vi "Organize new Comics.vi"() -> ()   [LabVIEW 2024]
uses:
  TypeDefs/comic--cluster.ctl
  TypeDefs/comics.reply--cluster.ctl
  <vilib>/addons/_JKI.lib/Serialization/JSON/JKI JSON Serialization.lvlib
panel:
  out "error out":errorcluster
  out "missing series":string[](array[string])
  out "current comic":string
  in  "comic repo path":path
  in  "comic data path":path
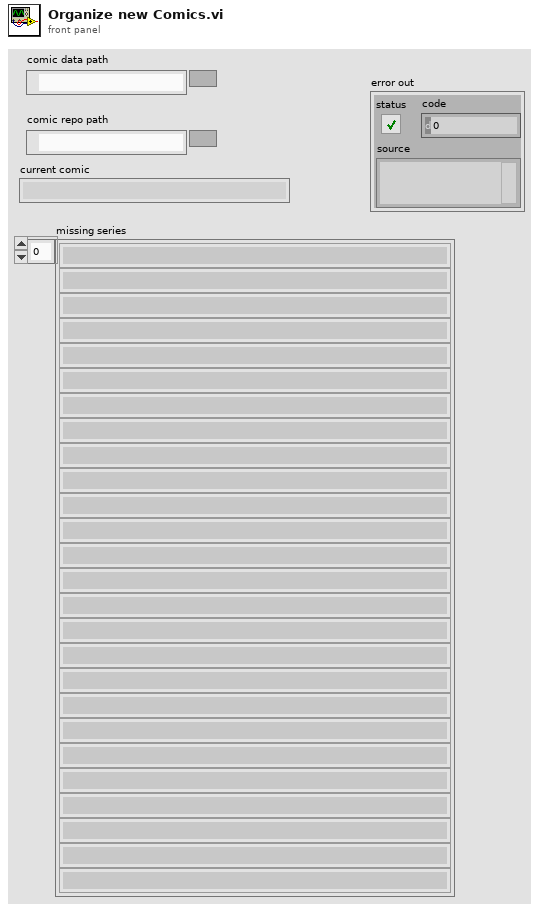
[diagram p1: front panel]
types:
  T1 = enum16{"open", "replace", "create", "open or create", "replace or create", "replace or create with confirmation"}
  T2 = typedef "comic--cluster.ctl" = cluster{"id":i32, "digitalId":i32, "title":string, "issueNumber":i32, "variantDescription":string, "description":string, "modified":variant, "upc":string, "format":string, "pageCount":i32, "resourceURI":string, "urls":cluster{"type":string, "url":string}[], "series":cluster{"resourceURI":string, "name":string}, "dates":cluster{"type":string, "date":string}[], "prices":cluster{"price":dbl, "type":string}[], "thumbnail":cluster{"path":string, "extension":string}, "images":cluster{"path":string, "extension":string}[], "creators":cluster{"available":i32, "returned":i32, "collectionURI":string, "items":cluster{"resourceURI":string, "name":string, "role":string}[]}, "characters":cluster{"available":i32, "returned":i32, "collectionURI":string, "items":cluster{"resourceURI":string, "name":string}[]}, "stories":cluster{"available":i32, "returned":i32, "collectionURI":string, "items":cluster{"resourceURI":string, "name":string, "type":string}[]}, "events":cluster{"available":i32, "returned":i32, "collectionURI":string, "items":cluster{"resourceURI":string, "name":string}[]}}
  T3 = typedef "comics.reply--cluster.ctl" = cluster{"code":i32, "status":string, "etag":string, "data":cluster{"offset":i32, "limit":i32, "total":i32, "count":i32, "results":T2[]}}
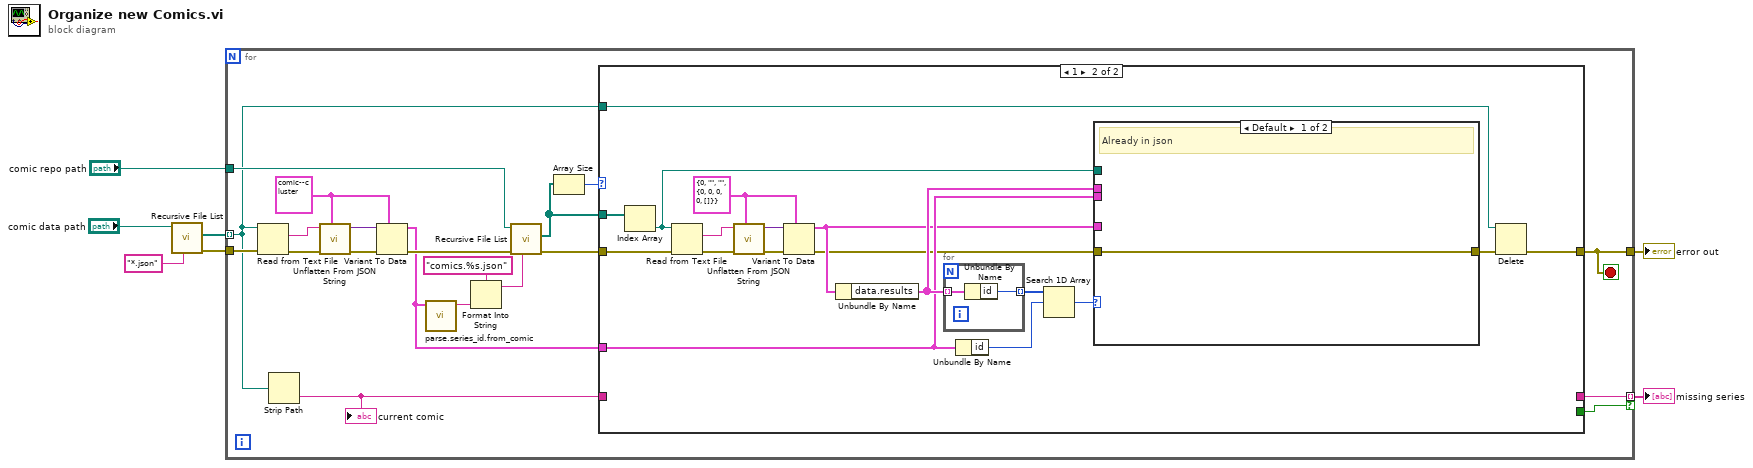
[diagram p0: block diagram]
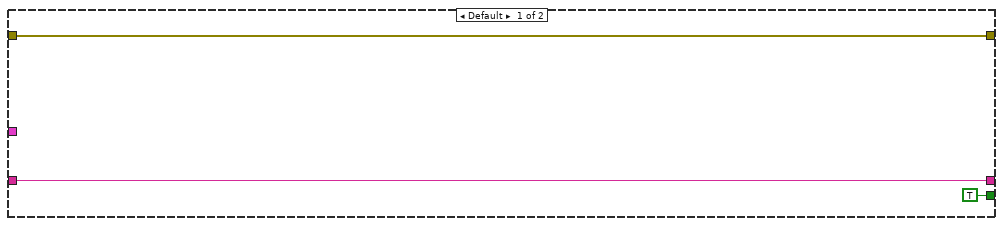
[diagram p2: hidden frame]
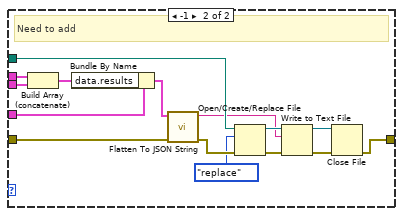
[diagram p3: hidden frame]
diagram:
  n1 = call <vilib>:"Recursive File List.vi"("pattern"="*.json", "Folder Path"="comic data path") -> ("error out"=w5:errorcluster, "All Files in Dir"=w6:path[])  [unwired: 5 in, 3 out]
  n2 = for {
    tunnel: w6 -> [w9] mode=indexing
    tunnel: w5 -> [w27]
    tunnel: "comic repo path" -> [w17]
    tunnel: [w14] -> w2 mode=indexing if=w13
    tunnel: [w8] -> w1
    stop <- w8 stop-if-true
    w22 = T2 {"id"=0, "digitalId"=0, "title"="", "issueNumber"=0, "variantDescription"="", "description"="", "modified"=variant, "upc"="", "format"="", "pageCount"=0, "resourceURI"="", "urls"=[], "series"={"resourceURI"="", "name"=""}, "dates"=[], "prices"=[], "thumbnail"={"path"="", "extension"=""}, "images"=[], "creators"={"available"=0, "returned"=0, "collectionURI"="", "items"=[]}, "characters"={"available"=0, "returned"=0, "collectionURI"="", "items"=[]}, "stories"={"available"=0, "returned"=0, "collectionURI"="", "items"=[]}, "events"={"available"=0, "returned"=0, "collectionURI"="", "items"=[]}} ("Cluster")
    n3 = Read from Text File(file (use dialog)=w9, error in=w27) -> (text=w25:string, error out=w26:errorcluster)  [unwired: 2 in, 2 out]
    n4 = Strip Path(path=w9) -> (name=w15:string)  [unwired: 1 out]
    "current comic" <- w15
    n5 = call <vilib>:"Unflatten From JSON String.vi"("Type and Defaults"=w22, "error in (no error)"=w26, "JSON String"=w25) -> ("error out"=w24:errorcluster, "Variant"=w23:variant)  [unwired: 7 in]
    n6 = Variant To Data(error in=w24, type=w22, Variant=w23) -> (data=w11:T2, error out=w21:errorcluster)
    n7 = call "parse.series_id.from_comic.vi"("comic"=w11) -> ("series_id"=w19:string)  [unwired: 10 in]
    n8 = Format Into String(format string="comics.%s.json", w19) -> (resulting string=w20:string)  [unwired: 2 in, 1 out]
    n9 = call <vilib>:"Recursive File List.vi"("pattern"=w20, "error in (no error)"=w21, "Folder Path"=w17) -> ("error out"=w10:errorcluster, "All Files in Dir"=w12:path[])  [unwired: 4 in, 3 out]
    n10 = Array Size(array=w12) -> (size(s)=w16:i32)
    n11 = case shown="1" w16 {
      tunnel: w15 -> [w28 _]
      tunnel: [w28 _] -> w14
      tunnel: [TRUE _] -> w13
      tunnel: w12 -> [_ w48]
      tunnel: w11 -> [_ w38]
      tunnel: w10 -> [w30 w35]
      tunnel: [w30 w33] -> w8
      tunnel: w9 -> [_ w31]
      frame Default {
      }
      frame 1 {
        w43 = T3 {"code"=0, "status"="", "etag"="", "data"={"offset"=0, "limit"=0, "total"=0, "count"=0, "results"=[]}} ("reply")
        n12 = Index Array(array=w48) -> (element=w34:path)  [unwired: 1 in]
        n13 = Read from Text File(file (use dialog)=w34, error in=w35) -> (text=w45:string, error out=w44:errorcluster)  [unwired: 2 in, 2 out]
        n14 = call <vilib>:"Unflatten From JSON String.vi"("Type and Defaults"=w43, "error in (no error)"=w44, "JSON String"=w45) -> ("error out"=w46:errorcluster, "Variant"=w47:variant)  [unwired: 7 in]
        n15 = Variant To Data(error in=w46, type=w43, Variant=w47) -> (data=w37:T3, error out=w36:errorcluster)
        n16 = Unbundle By Name(w37) -> ("data.results"=w39:T2[])
        n17 = for {
          tunnel: w39 -> [w66] mode=indexing
          tunnel: [w65] -> w42 mode=indexing
          n18 = Unbundle By Name(w66) -> ("id"=w65:i32)
        }
        n19 = Unbundle By Name(w38) -> ("id"=w41:i32)
        n20 = Search 1D Array(1D array=w42, element=w41) -> (index of element=w40:i32)  [unwired: 1 in]
        n21 = case shown="Default" w40 {
          tunnel: w39 -> [_ w64]
          tunnel: w38 -> [_ w63]
          tunnel: w37 -> [_ w62]
          tunnel: w36 -> [w49 w59]
          tunnel: w34 -> [_ w56]
          tunnel: [w49 w50] -> w32
          frame Default {
            # "Already in json"
          }
          frame -1 {
            # "Need to add"
            n22 = Build Array (concatenate)(w64, w63) -> (w61:T2[])
            n23 = Bundle By Name(cluster=w62, "data.results"=w61) -> (w60:T3)
            n24 = call <vilib>:"Flatten To JSON String.vi"("error in (no error)"=w59, "Variant"=w60) -> ("error out"=w58:errorcluster, "JSON String"=w53:string)  [unwired: 8 in]
            n25 = Open/Create/Replace File(file path (use dialog)=w56, error in=w58, operation (0:open)=T1."replace") -> (refnum out=w54:refnum<file>, error out=w55:errorcluster)  [unwired: 3 in, 1 out]
            n26 = Write to Text File(file (use dialog)=w54, text=w53, error in=w55) -> (refnum out=w51:refnum<file>, error out=w52:errorcluster)  [unwired: 1 in, 1 out]
            n27 = Close File(refnum=w51, error in=w52) -> (error out=w50:errorcluster)  [unwired: 1 out]
          }
        }
        n28 = Delete(path (use dialog)=w31, error in=w32) -> (error out=w33:errorcluster)  [unwired: 3 in, 2 out]
      }
    }
  }
  "missing series" <- w2
  "error out" <- w1
